vi "Write Command Core.vi"(8 "error in (no error)":errorcluster, 10 "Message":refnum<class "Message Interface.lvclass">, 11 "WS Client in":refnum<class "WS Client.lvclass">) -> (0 "error out":errorcluster, 2 "JSON String":string, 3 "WS Client out":refnum<class "WS Client.lvclass">)   [LabVIEW 2016, in "WebSocket Networking.lvlib" / "WS Client.lvclass"]
doc: "--\nCopyright © 2017 Composed SystemsI All rights reserved.\n\nAuthor: Jon McBee <jon.mcbee@composed.io>\n\nThis library is provided \"AS IS\" ,WITHOUT WARRANTIES OR\nCONDITIONS OF ANY KIND, either express or implied.\n\nComposed Systems -- composed.io\n\nStream 0.0.1.1\nJon McBee - Composed Systems\nCopyright (c) 2017, Composed Systems"
uses:
  <userlib>/Common Components/WebSocket Networking/WS Client/WS Client.lvclass
  <userlib>/Composed Systems/Stream/Mediator/Classes/Message Interface/Message Interface.lvclass
  <userlib>/Composed Systems/Stream/Mediator/Classes/Websocket Client Handler Actor/Websocket Client Handler/Websocket Client Handler.lvclass
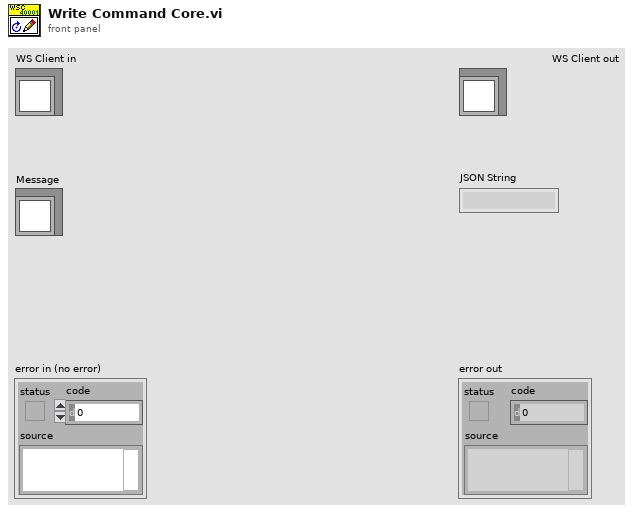
[diagram p1: front panel]
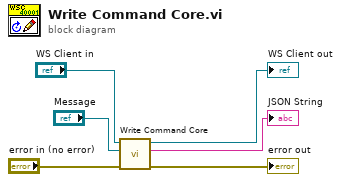
[diagram p0: block diagram]
diagram:
  n1 = call-parent "Write Command Core.vi"("error in (no error)"="error in (no error)", "Message"="Message", "Websocket Client Handler in"="WS Client in") -> ("error out"=→"error out":errorcluster, "JSON String"=→"JSON String":string, "Websocket Client Handler out"=→"WS Client out":refnum<class "WS Client.lvclass">)  [unwired: 6 in]
